vi "Helper-SubPanel.vi"() -> ()   [LabVIEW 2016]
uses:
  TypeDef/DataControl.ctl
panel:
  out "error out":errorcluster
  in  "error in":errorcluster
  in  "Stop":bool
  in  "Load SP2":bool
  in  "Load SP1":bool
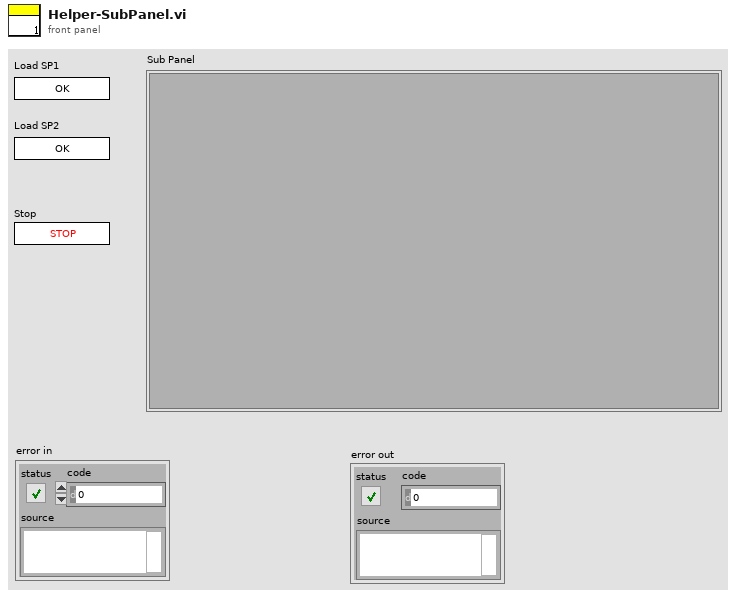
[diagram p1: front panel]
types:
  T1 = typedef "DataControl.ctl" = cluster{"SP no":i32, "Vi reference":refnum<vi>[]}
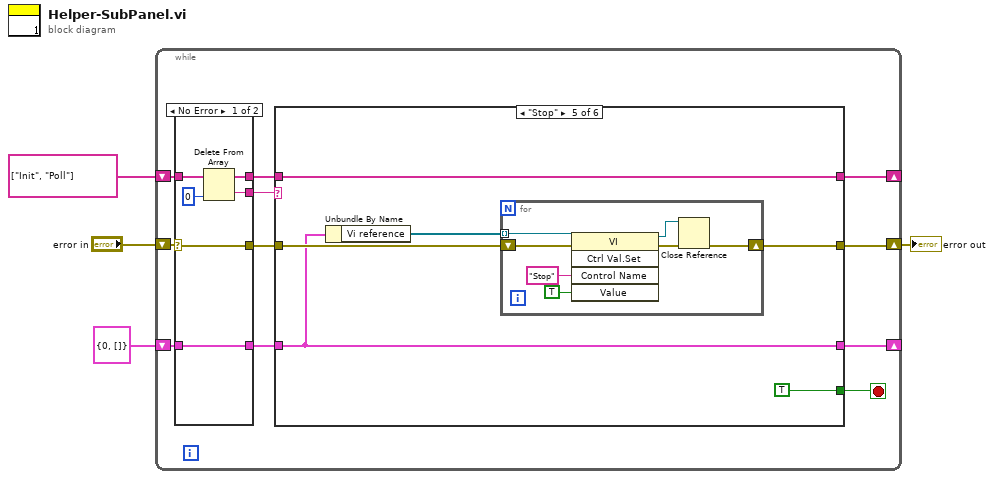
[diagram p0: block diagram]
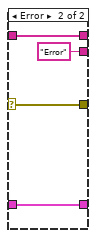
[diagram p2: hidden frame]
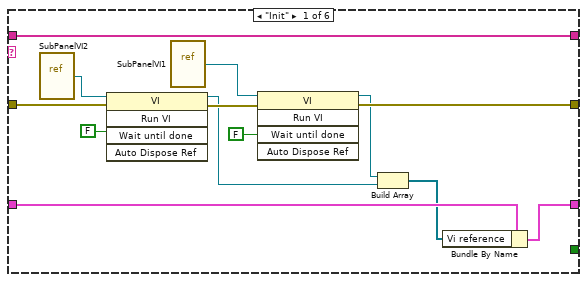
[diagram p3: hidden frame]
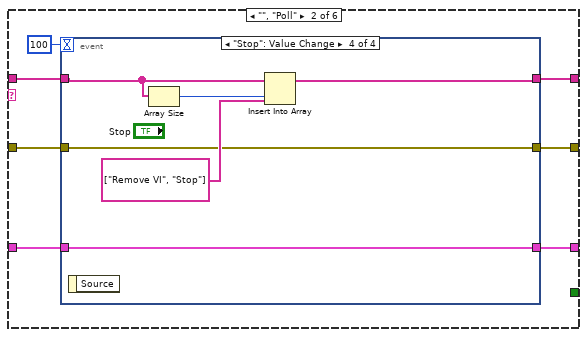
[diagram p4: hidden frame]
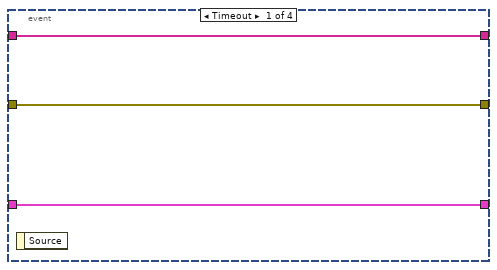
[diagram p5: hidden frame]
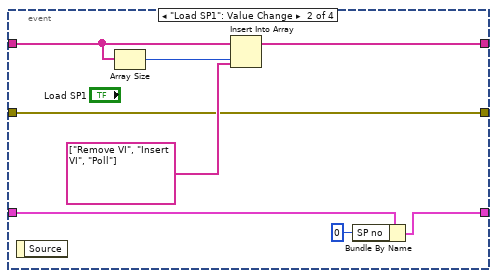
[diagram p6: hidden frame]
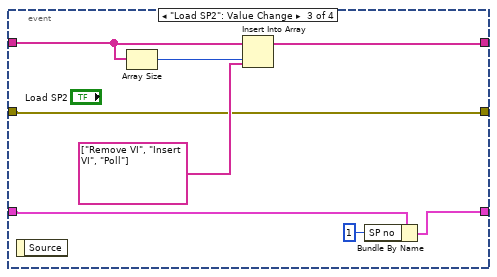
[diagram p7: hidden frame]
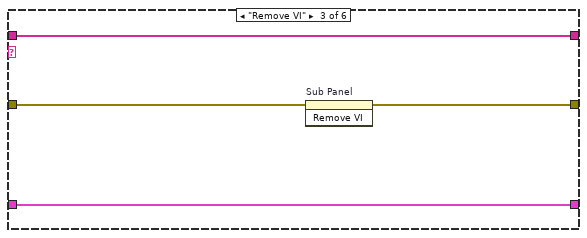
[diagram p8: hidden frame]
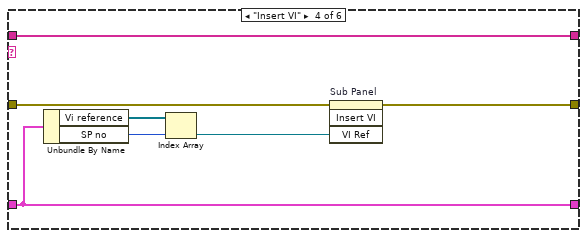
[diagram p9: hidden frame]
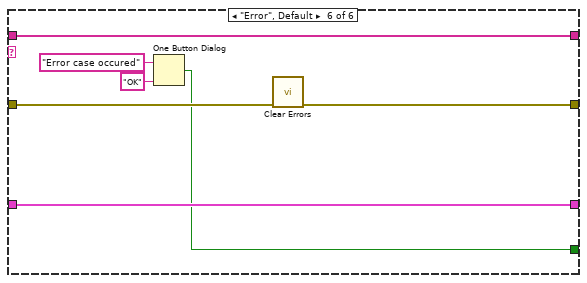
[diagram p10: hidden frame]
diagram:
  n1 = while {
    shift-right: [w14] -> _
    shift-left: string[] ["Init", "Poll"] -> [w15]
    shift-right: [w10] -> w1
    shift-left: "error in" -> [w12]
    shift-right: [w8] -> _
    shift-left: T1 {"SP no"=0, "Vi reference"=[]} -> [w7]
    stop <- w5 stop-if-true
    n2 = case shown="No Error" w12 {
      selector: w12 -> [w17 w23]
      tunnel: w15 -> [w21 w25]
      tunnel: [w20 w25] -> w13
      tunnel: [w18 "Error" ("String")] -> w9
      tunnel: [w17 w23] -> w11
      tunnel: w7 -> [w16 w22]
      tunnel: [w16 w22] -> w6
      frame No Error {
        n3 = Delete From Array(array=w21, index=0) -> (deleted portion=w18:string, array with subset deleted=w20:string[])  [unwired: 1 in]
      }
      frame Error {
      }
    }
    n4 = case shown="\"Stop\"" w9 {
      tunnel: [w38 w43 w74 w81 w87 w100] -> w14
      tunnel: w13 -> [w38 w44 w74 w81 w87 w100]
      tunnel: w11 -> [w34 w42 w71 w80 w84 w101]
      tunnel: [w35 w41 w72 w78 w85 w98] -> w10
      tunnel: [w29 w39 w73 w79 w83 w99] -> w8
      tunnel: w6 -> [w30 w40 w73 w79 w83 w99]
      tunnel: [_ _ _ _ TRUE w95] -> w5
      frame "Init" {
        n5 = vi-ref "SubPanelVI2.vi"() -> (w26:refnum<vi>)
        n6 = invoke class="VI" method="Run VI"(reference=w26, error in=w34, "Wait until done"=FALSE ("Wait Until Done")) -> (reference out=w31:refnum<vi>, error out=w33:errorcluster)  [unwired: 2 in, 3 out]
        n7 = vi-ref "SubPanelVI1.vi"() -> (w27:refnum<vi>)
        n8 = invoke class="VI" method="Run VI"(reference=w27, error in=w33, "Wait until done"=FALSE ("Wait Until Done")) -> (reference out=w32:refnum<vi>, error out=w35:errorcluster)  [unwired: 2 in, 3 out]
        n9 = Build Array(w32, w31) -> (w28:refnum<vi>[])
        n10 = Bundle By Name(cluster=w30, "Vi reference"=w28) -> (w29:T1)
      }
      frame "", "Poll" {
        n11 = event shown="[3] \"Stop\": Value Change" {
          selector: _ -> [_ _ _ _]
          dyn-events: _ -> [_ _ _ _]
          timeout: 100 -> [_ _ _ _]
          tunnel: w44 -> [w48 w54 w61 w69]
          tunnel: [w48 w55 w59 w68] -> w43
          tunnel: w42 -> [w47 w49 w60 w66]
          tunnel: [w47 w49 w60 w66] -> w41
          tunnel: w40 -> [w46 w52 w58 w65]
          tunnel: [w46 w51 w57 w65] -> w39
          event Timeout {
            n12 = event-data() -> ()  [unwired: 1 in, 1 out]
          }
          event "Load SP1": Value Change {
            n13 = event-data() -> ()  [unwired: 1 in, 1 out]
            n14 = Array Size(array=w54) -> (size(s)=w53:i32)
            n15 = Insert Into Array(array=w54, index=w53, new element=string[] ["Remove VI", "Insert VI", "Poll"]) -> (w55:string[])
            n16 = Bundle By Name(cluster=w52, "SP no"=0) -> (w51:T1)
          }
          event "Load SP2": Value Change {
            n17 = event-data() -> ()  [unwired: 1 in, 1 out]
            n18 = Array Size(array=w61) -> (size(s)=w63:i32)
            n19 = Insert Into Array(array=w61, index=w63, new element=string[] ["Remove VI", "Insert VI", "Poll"]) -> (w59:string[])
            n20 = Bundle By Name(cluster=w58, "SP no"=1) -> (w57:T1)
          }
          event "Stop": Value Change {
            n21 = event-data() -> ()  [unwired: 1 in, 1 out]
            n22 = Array Size(array=w69) -> (size(s)=w70:i32)
            n23 = Insert Into Array(array=w69, index=w70, new element=string[] ["Remove VI", "Stop"] ("new element/subarray")) -> (w68:string[])
          }
        }
      }
      frame "Remove VI" {
        n24 = invoke on="Sub Panel" class="SubPnl" method="Remove VI"(error in=w71) -> (error out=w72:errorcluster)  [unwired: 2 in, 2 out]
      }
      frame "Insert VI" {
        n25 = Unbundle By Name(w79) -> ("Vi reference"=w76:refnum<vi>[], "SP no"=w77:i32)
        n26 = Index Array(array=w76, index=w77) -> (element=w75:refnum<vi>)
        n27 = invoke on="Sub Panel" class="SubPnl" method="Insert VI"(error in=w80, "VI Ref"=w75) -> (error out=w78:errorcluster)  [unwired: 2 in, 3 out]
      }
      frame "Stop" {
        n28 = Unbundle By Name(w83) -> ("Vi reference"=w82:refnum<vi>[])
        n29 = for {
          shift-right: [w91] -> w85
          shift-left: w84 -> [w90]
          tunnel: w82 -> [w89] mode=indexing
          n30 = invoke class="VI" method="Ctrl Val.Set"(reference=w89, error in=w90, "Control Name"="Stop", "Value"=TRUE) -> (reference out=w88:refnum<vi>, error out=w92:errorcluster)  [unwired: 1 in, 3 out]
          n31 = Close Reference(reference=w88, error in (no error)=w92) -> (error out=w91:errorcluster)
        }
      }
      frame "Error", Default {
        n32 = One Button Dialog(message="Error case occured", button name ("OK")="OK") -> (true=w95:bool)
        n33 = call <vilib>:"Clear Errors.vi"("error in (no error)"=w101) -> ("error out"=w98:errorcluster)  [unwired: 5 in, 1 out]
      }
    }
  }
  "error out" <- w1
